vi "Visualize_Signals64.vi"(7 "FPGSampleTime":dbl=0.001500000013038516, 10 "tstart":dbl=-11.0, 11 "Signals":dbl[][](array[numeric])) -> (2 "plot(Signals) 33-64":T1, 3 "plot(Signals) 1-32":T2)   [LabVIEW 2014]
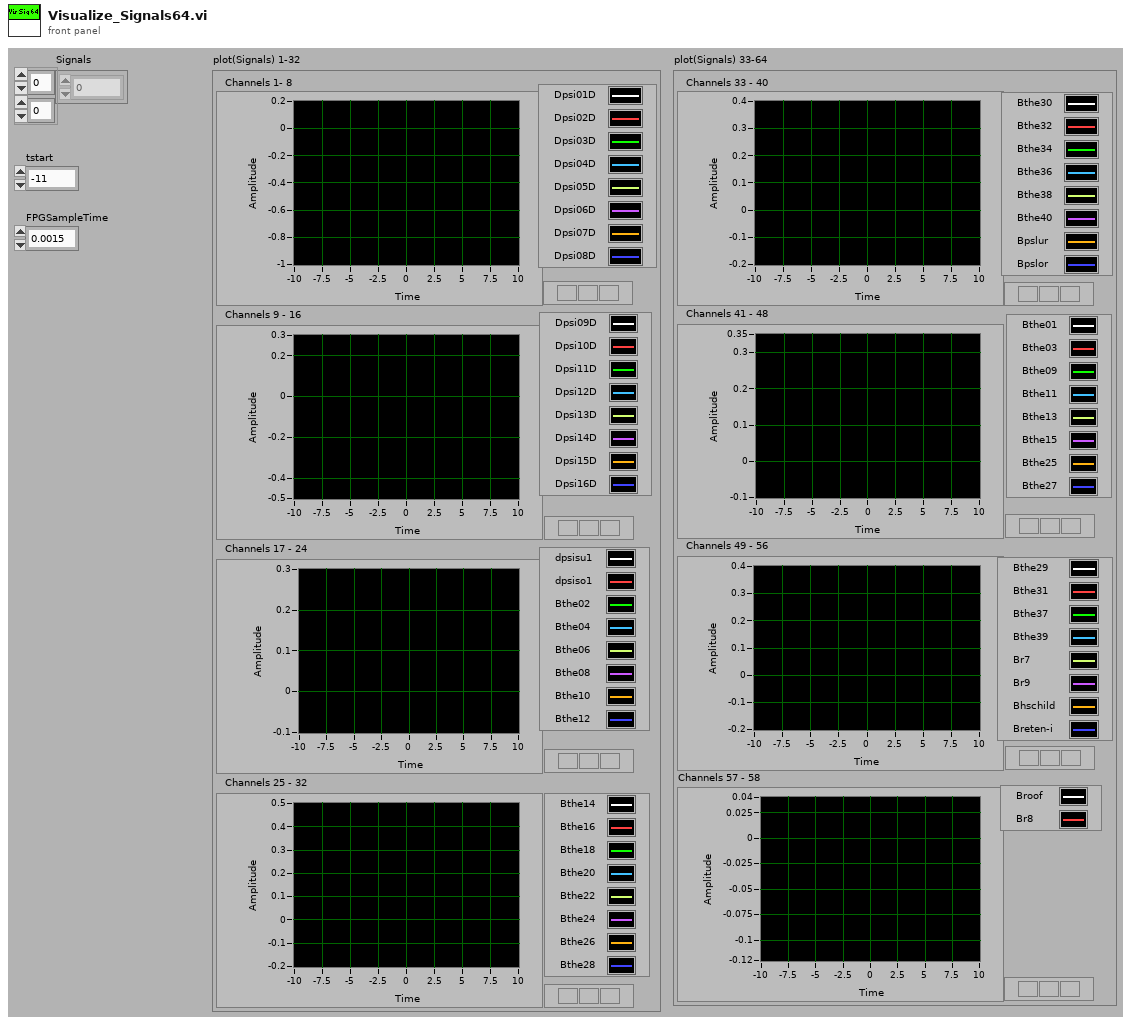
[diagram p1: front panel]
types:
  T1 = cluster{"Channels 33 - 40":cluster{"tstart":dbl, "FPGSampleTime":dbl, dbl[][]}, "Channels 41 - 48":cluster{"tstart":dbl, "FPGSampleTime":dbl, dbl[][]}, "Channels 49 - 56":cluster{"tstart":dbl, "FPGSampleTime":dbl, dbl[][]}, "Channels 57 - 58":cluster{"tstart":dbl, "FPGSampleTime":dbl, dbl[][]}}
  T2 = cluster{"Channels 1- 8":cluster{"tstart":dbl, "FPGSampleTime":dbl, dbl[][]}, "Channels 9 - 16":cluster{"tstart":dbl, "FPGSampleTime":dbl, dbl[][]}, "Channels 17 - 24":cluster{"tstart":dbl, "FPGSampleTime":dbl, dbl[][]}, "Channels 25 - 32":cluster{"tstart":dbl, "FPGSampleTime":dbl, dbl[][]}}
  T3 = cluster{"tstart":dbl, "FPGSampleTime":dbl, dbl[][]}
  T4 = cluster{cluster{"tstart":dbl, "FPGSampleTime":dbl, dbl[][]}, cluster{"tstart":dbl, "FPGSampleTime":dbl, dbl[][]}, cluster{"tstart":dbl, "FPGSampleTime":dbl, dbl[][]}, cluster{"tstart":dbl, "FPGSampleTime":dbl, dbl[][]}}
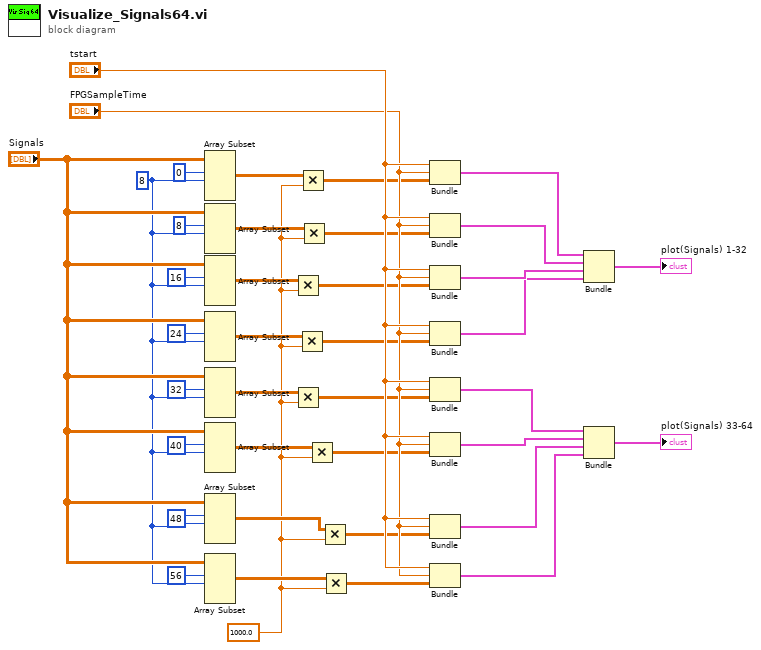
[diagram p0: block diagram]
diagram:
  w1 = 1000.0 ("y")
  w18 = 8 ("length")
  n1 = Array Subset(array="Signals", index (row)=0 ("index"), length (row)=w18) -> (w11:dbl[][])  [unwired: 2 in]
  n2 = Array Subset(array="Signals", index (row)=8 ("index"), length (row)=w18) -> (w3:dbl[][])  [unwired: 2 in]
  n3 = Array Subset(array="Signals", index (row)=16 ("index"), length (row)=w18) -> (w10:dbl[][])  [unwired: 2 in]
  n4 = Array Subset(array="Signals", index (row)=24 ("index"), length (row)=w18) -> (w9:dbl[][])  [unwired: 2 in]
  n5 = Array Subset(array="Signals", index (row)=32 ("index"), length (row)=w18) -> (w7:dbl[][])  [unwired: 2 in]
  n6 = Array Subset(array="Signals", index (row)=40 ("index"), length (row)=w18) -> (w5:dbl[][])  [unwired: 2 in]
  n7 = Array Subset(array="Signals", index (row)=48 ("index"), length (row)=w18) -> (w15:dbl[][])  [unwired: 2 in]
  n8 = Array Subset(array="Signals", index (row)=56 ("index"), length (row)=w18) -> (w17:dbl[][])  [unwired: 2 in]
  n9 = Multiply(x=w10, y=w1) -> (x*y=w13:dbl[][])
  n10 = Multiply(x=w7, y=w1) -> (x*y=w6:dbl[][])
  n11 = Multiply(x=w9, y=w1) -> (x*y=w8:dbl[][])
  n12 = Multiply(x=w11, y=w1) -> (x*y=w12:dbl[][])
  n13 = Multiply(x=w3, y=w1) -> (x*y=w2:dbl[][])
  n14 = Multiply(x=w5, y=w1) -> (x*y=w4:dbl[][])
  n15 = Multiply(x=w15, y=w1) -> (x*y=w14:dbl[][])
  n16 = Multiply(x=w17, y=w1) -> (x*y=w16:dbl[][])
  n17 = Bundle("tstart"="tstart", "FPGSampleTime"="FPGSampleTime", w12) -> (w29:T3)  [unwired: 1 out]
  n18 = Bundle("tstart"="tstart", "FPGSampleTime"="FPGSampleTime", w2) -> (w28:T3)  [unwired: 1 out]
  n19 = Bundle("tstart"="tstart", "FPGSampleTime"="FPGSampleTime", w13) -> (w27:T3)  [unwired: 1 out]
  n20 = Bundle("tstart"="tstart", "FPGSampleTime"="FPGSampleTime", w8) -> (w26:T3)  [unwired: 1 out]
  n21 = Bundle("tstart"="tstart", "FPGSampleTime"="FPGSampleTime", w6) -> (w24:T3)  [unwired: 1 out]
  n22 = Bundle("tstart"="tstart", "FPGSampleTime"="FPGSampleTime", w4) -> (w23:T3)  [unwired: 1 out]
  n23 = Bundle("tstart"="tstart", "FPGSampleTime"="FPGSampleTime", w14) -> (w22:T3)  [unwired: 1 out]
  n24 = Bundle("tstart"="tstart", "FPGSampleTime"="FPGSampleTime", w16) -> (w21:T3)  [unwired: 1 out]
  n25 = Bundle(w29, w28, w27, w26) -> (→"plot(Signals) 1-32":T4)  [unwired: 1 out]
  n26 = Bundle(w24, w23, w22, w21) -> (→"plot(Signals) 33-64":T4)  [unwired: 1 out]
